vi "4155C Make Big 2d array.vi"(0 "1D Var1":dbl[](array[numeric])=[0.0, 1.0, 2.0, 3.0, 4.0, 5.0, 6.0, 7.0, 8.0, 9.0, 10.0, 11.0] format="%.2f", 2 "1d IS":dbl[](array[numeric])=[20.0, 21.0, 22.0, 23.0, 24.0, 25.0, 26.0, 27.0, 28.0, 29.0, 30.0, 31.0] format="%.2f", 4 "1d ID":dbl[](array[numeric])=[40.0, 41.0, 42.0, 43.0, 44.0, 45.0, 46.0, 47.0, 48.0, 49.0, 50.0, 51.0] format="%.2f", 6 "1d IG":dbl[](array[numeric])=[60.0, 61.0, 62.0, 63.0, 64.0, 65.0, 66.0, 67.0, 68.0, 69.0, 70.0, 71.0] format="%.2f", 7 "1d SMU4":dbl[](array[numeric])=[60.0, 61.0, 62.0, 63.0, 64.0, 65.0, 66.0, 67.0, 68.0, 69.0, 70.0, 71.0] format="%.2f", 9 "SMU4":cluster{"on/off":bool, "Voltage":dbl} {"Voltage" min=-100.0 max=100.0 format="%.2f"}, 10 "VAR2 START":dbl format="%.2f", 11 "Number of VAR2 steps":i32=6, 14 "VAR2 STEP":dbl format="%.2f", 15 "VAR1 Name":string, 24 "Decimal places in header":i8=1, 26 "VAR2 Name":string) -> (20 "Header array":string[](array[string]), 22 "Data array":dbl[][](array[numeric]) format="%.2f")   [LabVIEW 2019]
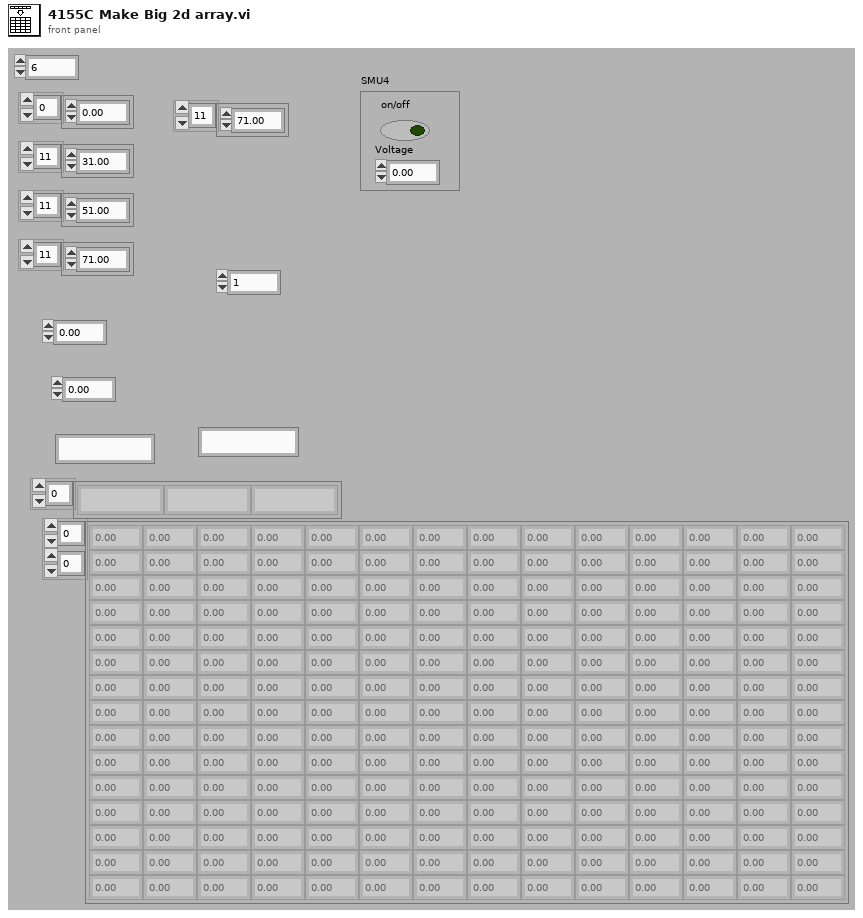
[diagram p1: front panel]
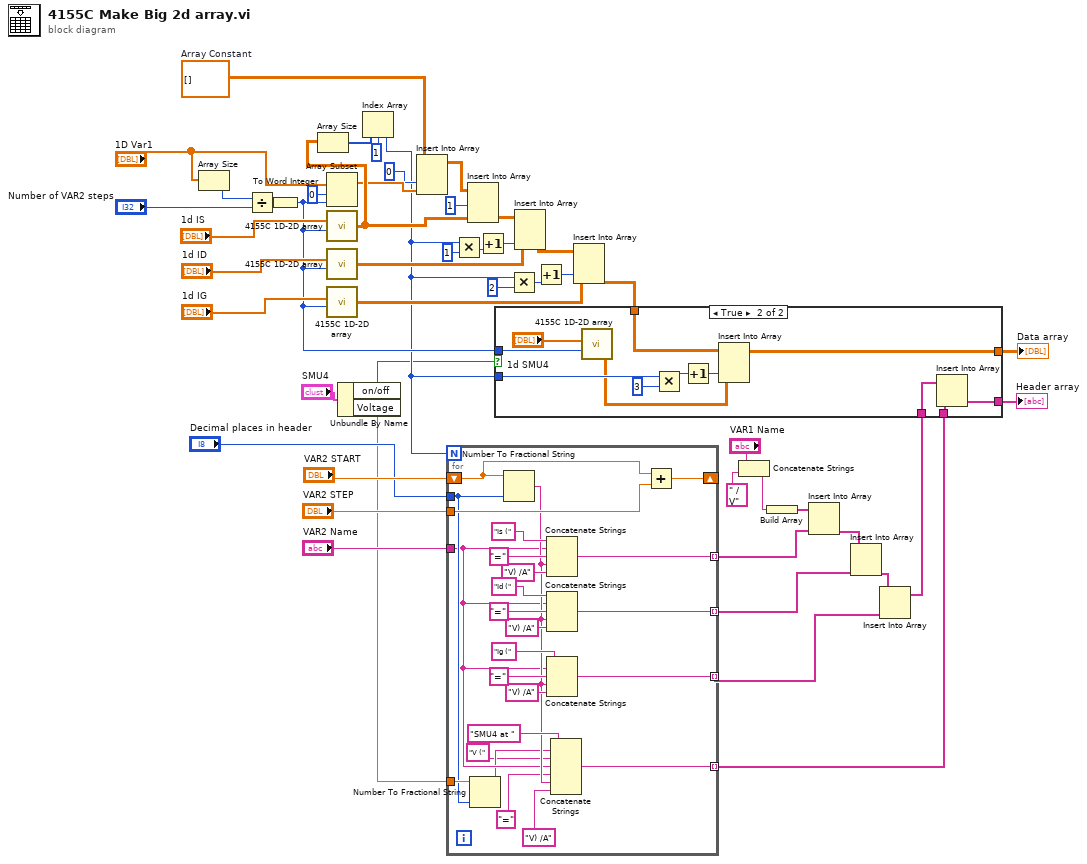
[diagram p0: block diagram]
diagram:
  w35 = dbl[][] []  # Array Constant
  n1 = Array Size(array="1D Var1") -> (size(s)=w12:i32)
  n2 = Divide(x=w12, y="Number of VAR2 steps") -> (x/y=w14:dbl)
  n3 = To Word Integer(number=w14) -> (16bit integer=w5:i16)
  n4 = Array Subset(array="1D Var1", index=0 ("Array Index"), length=w5) -> (w34:dbl[])
  n5 = call "4155C 1D-2D array.vi"("Number of VAR1 steps"=w5, "1D array in"="1d IS") -> ("2D array out"=w41:dbl[][])  [unwired: 4 in]
  n6 = Array Size(array=w41) -> (size(s)=w49:i32[])
  n7 = call "4155C 1D-2D array.vi"("Number of VAR1 steps"=w5, "1D array in"="1d ID") -> ("2D array out"=w45:dbl[][])  [unwired: 4 in]
  n8 = call "4155C 1D-2D array.vi"("Number of VAR1 steps"=w5, "1D array in"="1d IG") -> ("2D array out"=w42:dbl[][])  [unwired: 4 in]
  n9 = Unbundle By Name("SMU4") -> ("on/off"=w2:bool, "Voltage"=w1:dbl)
  n10 = Index Array(array=w49, index=1 ("Index")) -> (element=w4:i32)
  n11 = Insert Into Array(array=w35, index (col)=0 ("Disabled Index (col)"), new element=w34) -> (w36:dbl[][])  [unwired: 1 in]
  n12 = for {
    N: w4 -> [_]
    shift-right: [w74] -> _
    shift-left: "VAR2 START" -> [w73]
    tunnel: "VAR2 STEP" -> [w72]
    tunnel: "VAR2 Name" -> [w52]
    tunnel: [w69] -> w23 mode=indexing
    tunnel: [w62] -> w19 mode=indexing
    tunnel: [w61] -> w20 mode=indexing
    tunnel: "Decimal places in header" -> [w56]
    tunnel: [w58] -> w8 mode=indexing
    tunnel: w1 -> [w57]
    n13 = Number To Fractional String(number=w57, precision (6)=w56) -> (F-format string=w51:string)  [unwired: 2 in]
    n14 = Number To Fractional String(number=w73, precision (6)=w56) -> (F-format string=w54:string)  [unwired: 2 in]
    n15 = Concatenate Strings("Is (" ("Substring"), w52, "=" ("Substring"), w54, "V) /A" ("Substring")) -> (w69:string)
    n16 = Concatenate Strings("Id (" ("Substring"), w52, "=" ("Substring"), w54, "V) /A" ("Substring")) -> (w62:string)
    n17 = Concatenate Strings("Ig (" ("Substring"), w52, "=" ("Substring"), w54, "V) /A" ("Substring")) -> (w61:string)
    n18 = Concatenate Strings("SMU4 at " ("Substring"), w51, "V (" ("Substring"), w52, "=" ("Substring"), w54, "V) /A" ("Substring")) -> (w58:string)
    n19 = Add(x=w73, y=w72) -> (x+y=w74:dbl)
  }
  n20 = Multiply(x=w4, y=1) -> (x*y=w30:i32)
  n21 = Insert Into Array(array=w36, index (col)=1 ("Disabled Index (col)"), new element=w41) -> (w44:dbl[][])  [unwired: 1 in]
  n22 = Increment(x=w30) -> (x+1=w29:i32)
  n23 = Multiply(x=w4, y=2) -> (x*y=w31:i32)
  n24 = Insert Into Array(array=w44, index (col)=w29, new element=w45) -> (w43:dbl[][])  [unwired: 1 in]
  n25 = Increment(x=w31) -> (x+1=w28:i32)
  n26 = Insert Into Array(array=w43, index (col)=w28, new element=w42) -> (w10:dbl[][])  [unwired: 1 in]
  n27 = Concatenate Strings("VAR1 Name", " /V" ("Substring")) -> (w18:string)
  n28 = Build Array(w18) -> (w24:string[])
  n29 = Insert Into Array(array=w24, new element=w23) -> (w22:string[])  [unwired: 1 in]
  n30 = Insert Into Array(array=w22, new element=w19) -> (w21:string[])  [unwired: 1 in]
  n31 = Insert Into Array(array=w21, new element=w20) -> (w7:string[])  [unwired: 1 in]
  n32 = case shown="True" w2 {
    tunnel: w10 -> [w76 w82]
    tunnel: [w76 w80] -> w9
    tunnel: w8 -> [_ w78]
    tunnel: w7 -> [w75 w79]
    tunnel: [w75 w77] -> w6
    tunnel: w5 -> [_ w88]
    tunnel: w4 -> [_ w85]
    frame False {
    }
    frame True {
      n33 = call "4155C 1D-2D array.vi"("Number of VAR1 steps"=w88, "1D array in"="1d SMU4") -> ("2D array out"=w81:dbl[][])  [unwired: 4 in]
      n34 = Multiply(x=w85, y=3) -> (x*y=w84:i32)
      n35 = Increment(x=w84) -> (x+1=w83:i32)
      n36 = Insert Into Array(array=w82, index (col)=w83, new element=w81) -> (w80:dbl[][])  [unwired: 1 in]
      n37 = Insert Into Array(array=w79, new element=w78) -> (w77:string[])  [unwired: 1 in]
    }
  }
  "Data array" <- w9
  "Header array" <- w6
